vi "Null Broadcast Events--constant.vi"() -> (3 "DB_CONNECTOR Broadcast Events":T1)   [LabVIEW 2020, in "hse-db.lvlib" / "DB_CONNECTOR.lvlib"]
doc: "Returns the broadcast events cluster with null references for defining the event types in a Register For Events function.\n____\nHAMPEL SOFTWARE ENGINEERING v1.4.0 (2023-12-19 09:52)"
uses:
  DB_CONNECTOR.lvlib
  Broadcast Events--cluster.ctl
  Did Init Argument--cluster.ctl
  Status Updated Argument--cluster.ctl
  Error Reported Argument--cluster.ctl
  Stop Argument--cluster.ctl
  Get Module Execution Status Argument--cluster.ctl
  Fast Query Reply Argument--cluster.ctl
  Configured and Connected Argument--cluster.ctl
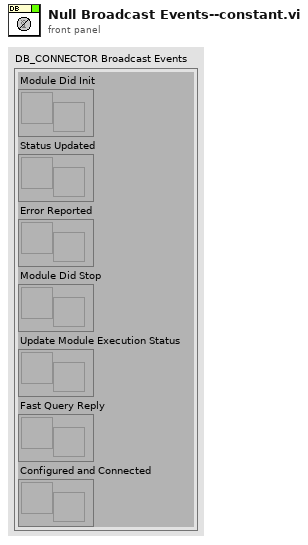
[diagram p1: front panel]
types:
  T1 = typedef "hse-db.lvlib/DB_CONNECTOR.lvlib/Broadcast Events--cluster.ctl" = cluster{"Module Did Init":refnum<user-event>, "Status Updated":refnum<user-event>, "Error Reported":refnum<user-event>, "Module Did Stop":refnum<user-event>, "Update Module Execution Status":refnum<user-event>, "Fast Query Reply":refnum<user-event>, "Configured and Connected":refnum<user-event>}
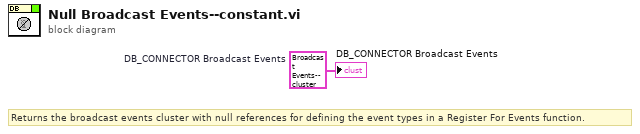
[diagram p0: block diagram]
diagram:
  w1 = T1 {"Module Did Init"=refnum, "Status Updated"=refnum, "Error Reported"=refnum, "Module Did Stop"=refnum, "Update Module Execution Status"=refnum, "Fast Query Reply"=refnum, "Configured and Connected"=refnum}  # DB_CONNECTOR Broadcast Events
  # "Returns the broadcast events cluster with null references for defining the event types in a Register For Events function."
  "DB_CONNECTOR Broadcast Events" <- w1
